vi "CalculateAsynchronous.vi"(6 "calc cache":variant, 7 "Feature":T1, 8 "error in (no error)":errorcluster, 9 "Speed (RPM)":dbl, 11 "Data":waveform(sgl)) -> (0 "error out":errorcluster, 3 "Asynchronous [EU RMS]":dbl, 4 "calc cache out":variant)   [LabVIEW 2017, in "AnalysisHelper.lvlib"]
uses:
  <vilib>/addons/InsightCM/Utilities/Analysis/Shared/AnalysisHelper.lvlib
  <vilib>/addons/InsightCM/Utilities/Analysis/Shared/controls/Feature.ctl
  <vilib>/addons/InsightCM/Utilities/Analysis/Shared/controls/AmplitudeScale.ctl
  <vilib>/addons/InsightCM/Utilities/Analysis/Vibration/VibrationAnalysisFunctions.lvlib
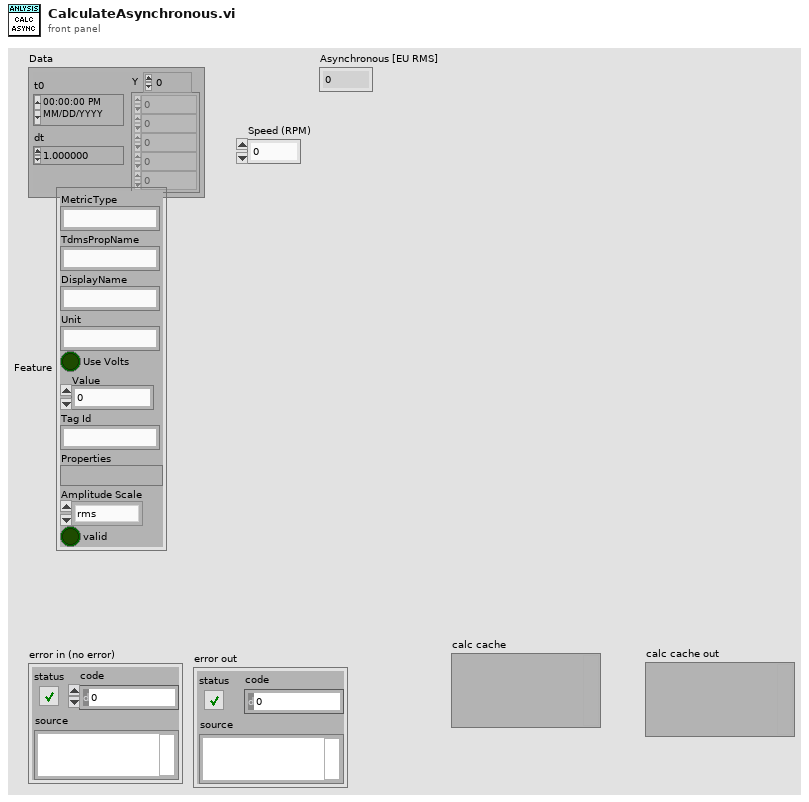
[diagram p1: front panel]
types:
  T1 = typedef "AnalysisHelper.lvlib/Feature.ctl" = cluster{"MetricType":string, "TdmsPropName":string, "DisplayName":string, "Unit":string, "Use Volts":bool, "Value":dbl, "Tag Id":string, "Properties":variant, "Amplitude Scale":T2, "valid":bool}
  T2 = typedef "AnalysisHelper.lvlib/AmplitudeScale.ctl" = enum16{"rms", "peak", "pk-pk"}
  T3 = typedef "svc_Spectrum Info.ctl" = cluster{"channel name":string, "description":string, "x-axis units":T4, "spectral info":cluster{"spectrum type":T5, "linear/dB":enum16{"linear", "dB"}, "window":u16, "window size":i32, "FFT size":i32}, "engineering units":T6, "custom label":string, "dB reference [EU]":dbl, "peak units":enum16{"rms", "peak", "peak-peak"}, "weighting filter":T7, "spectral density?":bool, "unit label":string, "spectrum skewed?":bool, "complimentary spectrum units":T8}
  T4 = typedef "svc_X-Axis Units.ctl" = u16
  T5 = typedef "svc_Spectrum Type.ctl" = enum16{"FFT Spectrum [complex]", "Amplitude [Magnitude]", "Power [Magnitude^2]", "Cross Spectrum [complex]", "Frequency Response [Complex]"}
  T6 = typedef "svc_Engineering Units Text Ring.ctl" = u16
  T7 = typedef "svc_Weighting Filter Text Ring.ctl" = u16
  T8 = typedef "svc_Complimentary Spectrum Units.ctl" = enum16{"none", "radians", "degrees", "cycles", "imaginary"}
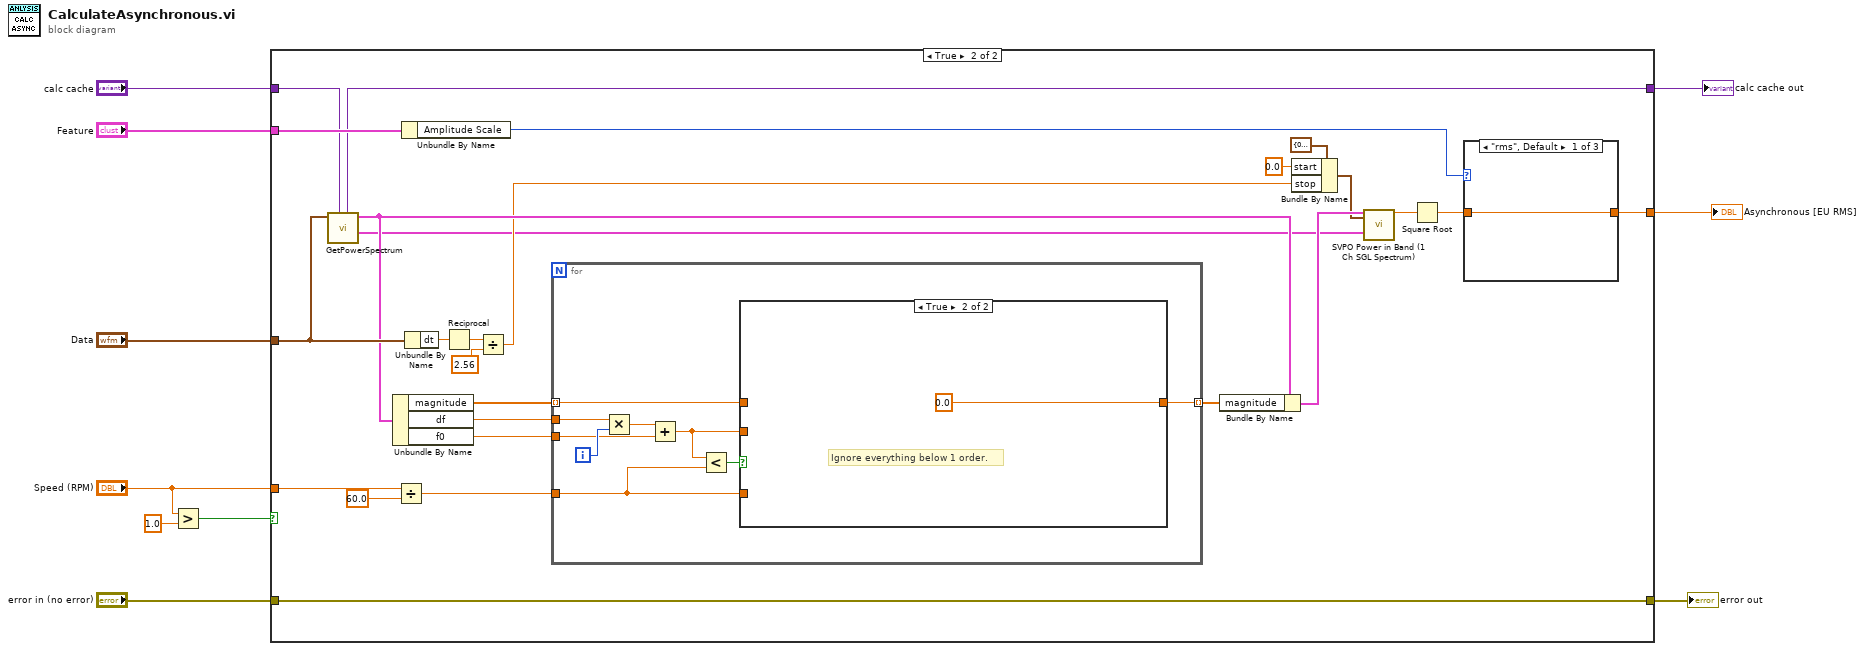
[diagram p0: block diagram]
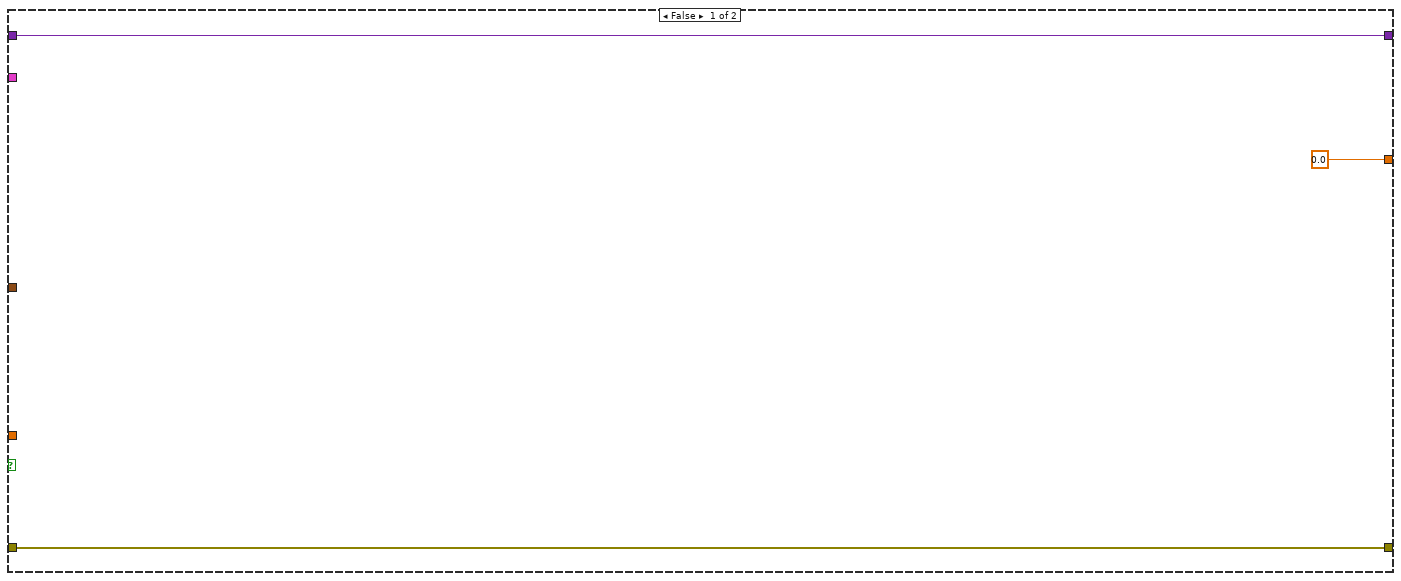
[diagram p2: hidden frame]
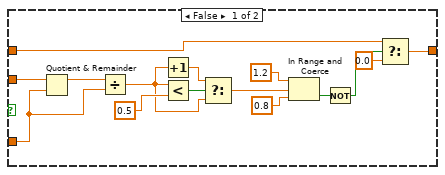
[diagram p3: hidden frame]
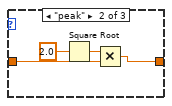
[diagram p4: hidden frame]
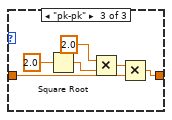
[diagram p5: hidden frame]
diagram:
  n1 = Greater?(x="Speed (RPM)", y=1.0) -> (0:w3:bool)
  n2 = case shown="True" w3 {
    tunnel: "Speed (RPM)" -> [_ w16]
    tunnel: "Data" -> [_ w38]
    tunnel: "error in (no error)" -> [w12 w28]
    tunnel: "Feature" -> [_ w27]
    tunnel: [0.0 w26] -> w7
    tunnel: "calc cache" -> [w11 w20]
    tunnel: [w12 w28] -> w5
    tunnel: [w11 w18] -> w1
    frame False {
    }
    frame True {
      n3 = call <vilib>:"GetPowerSpectrum.vi"("calc cache"=w20, "Waveform"=w38) -> ("spectrum info"=w22:T3, "power spectrum [EU^2 rms]"=w34:cluster{"f0":dbl, "df":dbl, "magnitude":sgl[]}, "calc cache out"=w18:variant)  [unwired: 7 in]
      n4 = Unbundle By Name(w34) -> ("magnitude"=w32:sgl[], "df"=w39:dbl, "f0"=w17:dbl)
      n5 = Divide(x=w16, y=60.0) -> (x/y=w14:dbl)
      n6 = Unbundle By Name(w27) -> ("Amplitude Scale"=w25:T2)
      n7 = Unbundle By Name(w38) -> ("dt"=w37:dbl)
      n8 = Reciprocal(x=w37) -> (1/x=w36:dbl)
      n9 = Divide(x=w36, y=2.56) -> (x/y=w29:dbl)
      n10 = for {
        tunnel: w32 -> [w41] mode=indexing
        tunnel: w39 -> [w48]
        tunnel: w17 -> [w46]
        tunnel: w14 -> [w40]
        tunnel: [w43] -> w33 mode=indexing
        i -> [w47]
        n11 = Multiply(x=w48, y=w47) -> (x*y=w45:dbl)
        n12 = Add(x=w45, y=w46) -> (x+y=w42:dbl)
        n13 = Less?(x=w42, y=w40) -> (x < y?=w44:bool)
        n14 = case shown="True" w44 {
          tunnel: [w52 sgl 0.0 ("y")] -> w43
          tunnel: w42 -> [w63 _]
          tunnel: w41 -> [w53 _]
          tunnel: w40 -> [w61 _]
          frame False {
            n15 = Quotient & Remainder(x=w63, y=w61) -> (x-y*floor(x/y)=w62:dbl)  [unwired: 1 out]
            n16 = Divide(x=w62, y=w61) -> (x/y=w57:dbl)
            n17 = Increment(x=w57) -> (x+1=w58:dbl)
            n18 = Less?(x=w57, y=0.5) -> (x < y?=w59:bool)
            n19 = Select(t=w58, s=w59, f=w57) -> (s? t:f=w54:dbl)
            n20 = In Range and Coerce(upper limit=1.2, x=w54, lower limit=0.8) -> (In Range?=w50:bool)  [unwired: 1 out]
            n21 = Not(x=w50) -> (.not. x?=w49:bool)
            n22 = Select(t=w53, s=w49, f=sgl 0.0) -> (s? t:f=w52:sgl)
          }
          frame True {
            # "Ignore everything below 1 order."
          }
        }
      }
      n23 = Bundle By Name(cluster=w34, "magnitude"=w33) -> (w24:cluster{"f0":dbl, "df":dbl, "magnitude":sgl[]})
      n24 = Bundle By Name(cluster=cluster{"start":dbl, "stop":dbl} {"start"=0.0, "stop"=1000.0} ("range"), "start"=0.0, "stop"=w29) -> (w23:cluster{"start":dbl, "stop":dbl})
      n25 = call <vilib>:"SVPO Power in Band (1 Ch SGL Spectrum).vi"("spectrum [EU^2 rms]"=w24, "range"=w23, "spectrum info"=w22) -> ("power in band [EU^2 rms]"=w21:dbl)  [unwired: 16 in]
      n26 = Square Root(x=w21) -> (sqrt(x)=w19:dbl)
      n27 = case shown="\"rms\", Default" w25 {
        tunnel: w19 -> [w65 w69 w75]
        tunnel: [w65 w68 w74] -> w26
        frame "rms", Default {
        }
        frame "peak" {
          n28 = Square Root(x=sgl 2.0) -> (sqrt(x)=w67:sgl)
          n29 = Multiply(x=w67, y=w69) -> (x*y=w68:dbl)
        }
        frame "pk-pk" {
          n30 = Square Root(x=sgl 2.0) -> (sqrt(x)=w71:sgl)
          n31 = Multiply(x=sgl 2.0, y=w71) -> (x*y=w72:sgl)
          n32 = Multiply(x=w72, y=w75) -> (x*y=w74:dbl)
        }
      }
    }
  }
  "Asynchronous [EU RMS]" <- w7
  "error out" <- w5
  "calc cache out" <- w1
